vi "CNTRLR - Wash Step Transform.vi"(8 "error in (no error)":errorcluster, 10 "Wash Step":string, 11 "View Model":T2) -> (0 "error out":errorcluster, 2 "Wash Step Enum":T1, 3 "View Model":T2)   [LabVIEW 2017]
doc: "Transforms current Wash Step from STR into TypeDef Enum."
uses:
  View Model/Controls/View Model.ctl
  View Model/Controls/Shared Model.ctl
  Error Handler/Controls/Error Model.ctl
  Error Handler/Controls/Error Message.ctl
  Error Handler/Controls/Error Level.ctl
  Configuration/Controls/Database Model.ctl
  Configuration/Controls/Database Message.ctl
  Configuration/Controls/Database Command.ctl
  Configuration/Controls/Database Overhead.ctl
  Configuration/Controls/Database Status.ctl
  Configuration/Controls/Database Record.ctl
  Configuration/Controls/Database - Rule Record.ctl
  Controls/CNTRLR - Wash Step.ctl
  Controls/CNTRLR - Position.ctl
  Controls/CNTRLR - Model.ctl
  Controls/CNTRLR - Message.ctl
  Controls/CNTRLR - Command.ctl
  Controls/CNTRLR - Overhead.ctl
  Controls/CNTRLR - State.ctl
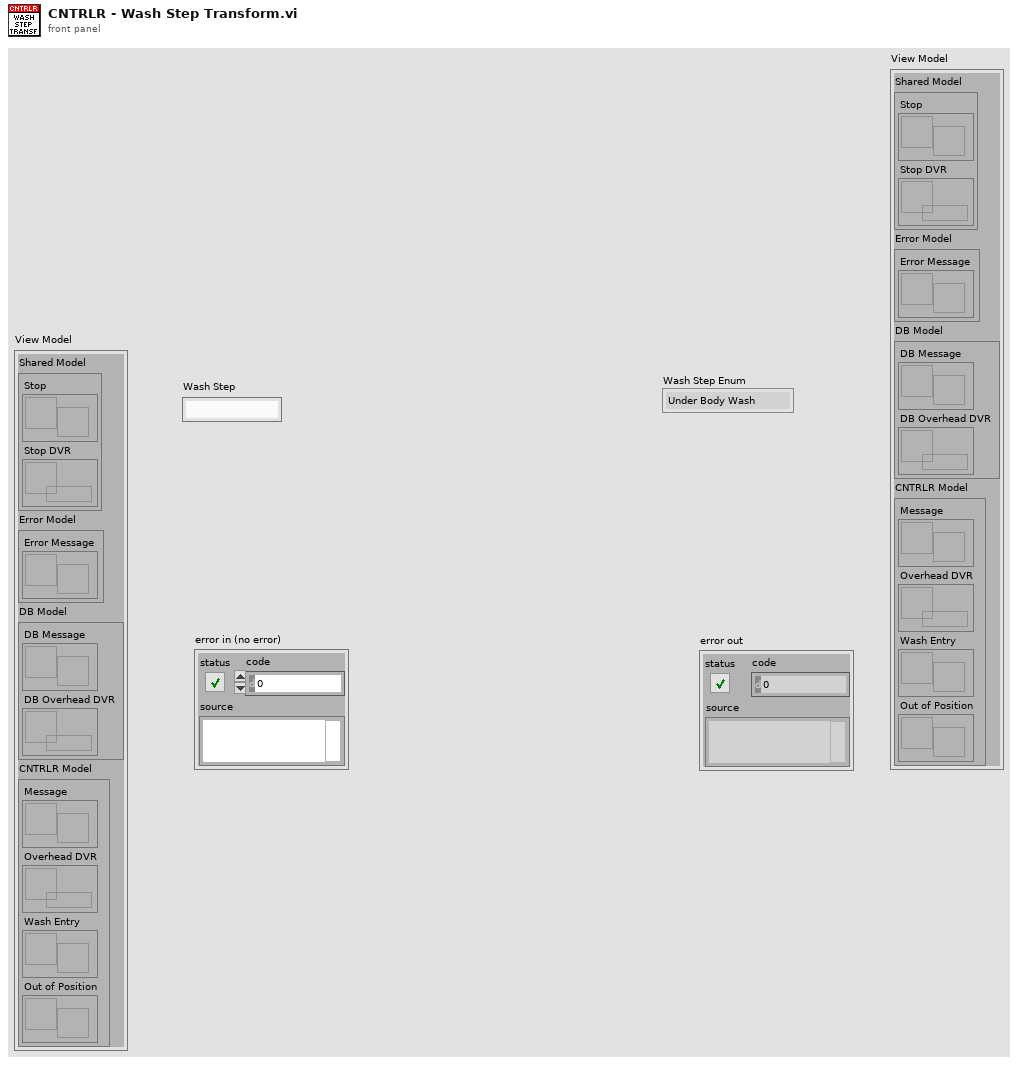
[diagram p1: front panel]
types:
  T1 = typedef "CNTRLR - Wash Step.ctl" = enum16{"Under Body Wash", "Bug Remover", "Pre-Soak", "High Pressure Wash", "Low Pressure Wax", "Spot Free Rinse", "Tire Shine Foam", "Air Dry", "None"}
  T2 = typedef "View Model.ctl" = cluster{"Shared Model":T3, "Error Model":T4, "DB Model":T5, "CNTRLR Model":T6}
  T3 = typedef "Shared Model.ctl" = cluster{"Stop":refnum<user-event>, "Stop DVR":refnum<data-value>}
  T4 = typedef "Error Model.ctl" = cluster{"Error Message":refnum<user-event>}
  T5 = typedef "Database Model.ctl" = cluster{"DB Message":refnum<user-event>, "DB Overhead DVR":refnum<data-value>}
  T6 = typedef "CNTRLR - Model.ctl" = cluster{"Message":refnum<user-event>, "Overhead DVR":refnum<data-value>, "Wash Entry":refnum<user-event>, "Out of Position":refnum<user-event>}
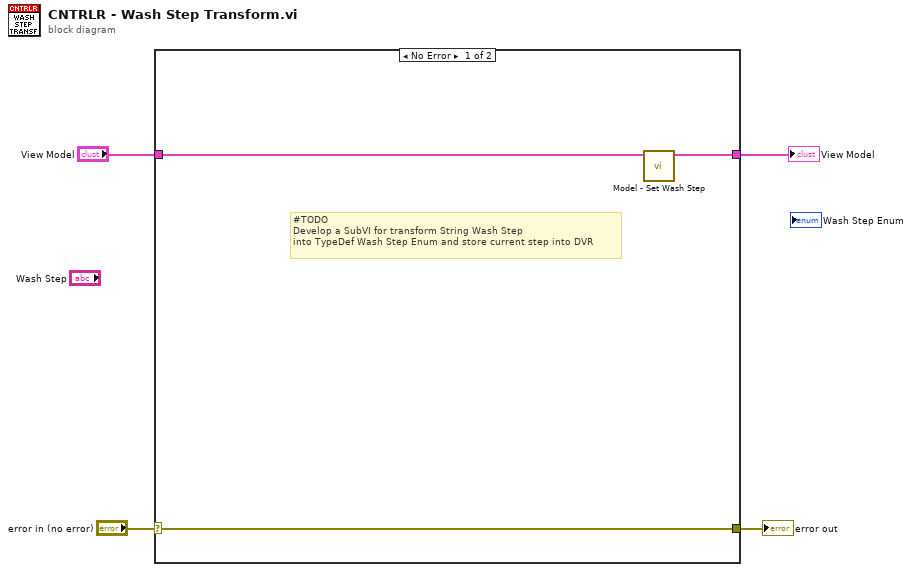
[diagram p0: block diagram]
diagram:
  n1 = case shown="No Error" "error in (no error)" {
    selector: "error in (no error)" -> [w7 w9]
    tunnel: [w7 w9] -> w3
    tunnel: "View Model" -> [w6 w8]
    tunnel: [w5 w8] -> w1
    frame No Error {
      # "#TODO\nDevelop a SubVI for transform String Wash Step\ninto TypeDef Wash Step Enum and store current step into DVR"
      n2 = call "Model - Set Wash Step.vi"("View Model"=w6) -> ("View Model"=w5:T2)  [unwired: 9 in, 1 out]
    }
    frame Error {
    }
  }
  "error out" <- w3
  "View Model" <- w1
